vi "Paddle move.vi"(5 "AreaSize":T1, 6 "Paddle Ref":refnum<vi>, 7 "offset":i32) -> (1 "Left":i32)   [LabVIEW 8.6]
uses:
  <vilib>/Utility/miscctls.llb/LVBoundsTypeDef.ctl
panel:
  out "Label.Text":string
  in  "Blank Button":bool
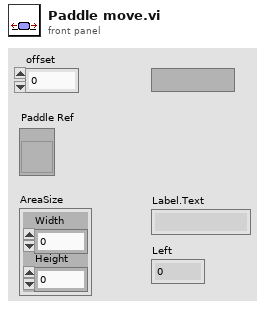
[diagram p1: front panel]
types:
  T1 = typedef "LVBoundsTypeDef.ctl" = cluster{"Width":u32, "Height":u32}
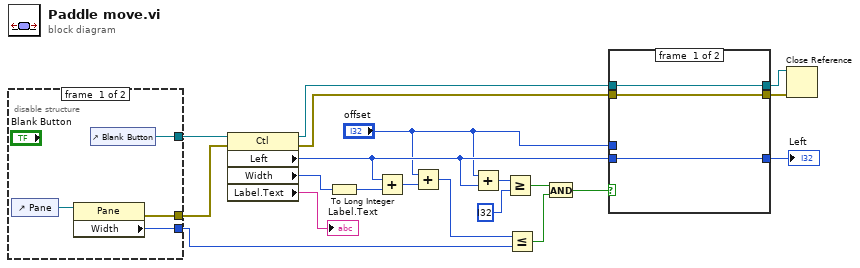
[diagram p0: block diagram]
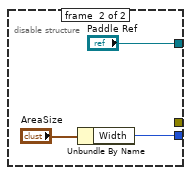
[diagram p2: hidden frame]
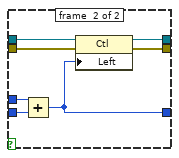
[diagram p3: hidden frame]
diagram:
  n1 = disable-structure shown="Enabled" {
    disable-tunnel: [w24 "Paddle Ref"] -> w19
    disable-tunnel: [w22 w25] -> w4
    disable-tunnel: [w21 _] -> w3
    frame #0 {
      n2 = control-ref of="Pane"() -> (w23:refnum<vi>)
      n3 = property class="Pane"(reference=w23) -> (error out=w21:errorcluster, "Width"=w22:u32)  [unwired: 1 in, 1 out]
      n4 = control-ref of="Blank Button"() -> (w24:refnum<vi>)
    }
    frame #1 {
      n5 = Unbundle By Name("AreaSize") -> ("Width"=w25:u32)
    }
  }
  n6 = property class="Ctl"(reference=w19, error in=w3) -> (reference out=w7:refnum<vi>, error out=w6:errorcluster, "Left"=w17:i32, "Width"=w20:u32, "Label.Text"=→"Label.Text":string)
  n7 = To Long Integer(number=w20) -> (32bit integer=w18:i32)
  n8 = Add(x=w17, y=w18) -> (x+y=w12:i32)
  n9 = Add(x="offset", y=w12) -> (x+y=w11:i32)
  n10 = Add(x="offset", y=w17) -> (x+y=w13:i32)
  n11 = Greater Or Equal?(x=w13, y=i32 ?) -> (x >= y?=w15:bool)
  n12 = Less Or Equal?(x=w11, y=w4) -> (x <= y?=w14:bool)
  n13 = And(x=w15, y=w14) -> (x .and. y?=w9:bool)
  n14 = case shown="True" w9 {
    tunnel: "offset" -> [_ w37]
    tunnel: w17 -> [w30 w36]
    tunnel: [w30 w35] -> w10
    tunnel: w7 -> [w29 w34]
    tunnel: w6 -> [w28 w33]
    tunnel: [w29 w32] -> w2
    tunnel: [w28 w31] -> w1
    frame #0 {
    }
    frame #1 {
      n15 = Add(x=w37, y=w36) -> (x+y=w35:i32)
      n16 = property class="Ctl"(reference=w34, error in=w33, "Left"=w35) -> (reference out=w32:refnum<vi>, error out=w31:errorcluster)
    }
  }
  "Left" <- w10
  n17 = Close Reference(reference=w2, error in (no error)=w1) -> ()  [unwired: 1 out]
